vi "UnregisterForDiagPackets.vi"(8 "error in (no error)":errorcluster, 9 "Even Metadata":T1) -> (0 "error out":errorcluster)   [LabVIEW 2013]
uses:
  C:/GEECS/Developers Version/source/Device Driver/AerotechStage/Sample Vis/Bin/Aerotech.Ensemble.LabVIEW.dll
  Bin/Aerotech.Ensemble.LabVIEW.dll
  ControllerDiagPacket.ctl
  AxisDiagPacket.ctl
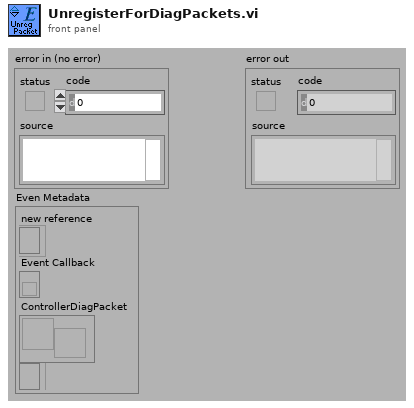
[diagram p1: front panel]
types:
  T1 = cluster{"new reference":refnum<k24>, "Event Callback":refnum<k27>, "ControllerDiagPacket":refnum<user-event>, "Event Registration Refnum":refnum<event-registration>}
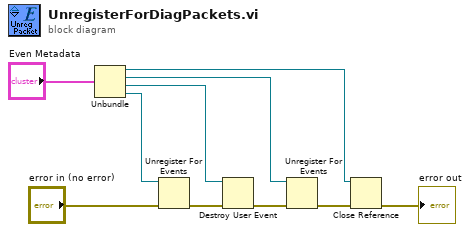
[diagram p0: block diagram]
diagram:
  n1 = Unbundle("Even Metadata") -> ("new reference"=w2:refnum<k24>, "Event Callback"=w5:refnum<k27>, "ControllerDiagPacket"=w6:refnum<user-event>, "Event Registration Refnum"=w7:refnum<event-registration>)
  n2 = Unregister For Events(event registration refnum=w7, error in="error in (no error)") -> (error out=w9:errorcluster)
  n3 = Destroy User Event(user event=w6, error in=w9) -> (error out=w8:errorcluster)
  n4 = Unregister For Events(event registration refnum=w5, error in=w8) -> (error out=w4:errorcluster)
  n5 = Close Reference(reference=w2, error in (no error)=w4) -> (error out=→"error out":errorcluster)
